vi "DiJian_1.vi"(8 "error in":errorcluster, 10 "地检1相位":i32, 11 "VISA资源名称":refnum<visa-resource-name>) -> (0 "错误输出":errorcluster, 2 "地检1相位输出":i32, 3 "VISA资源名称输出":refnum<visa-resource-name>)   [LabVIEW 2012]
uses:
  <vilib>/GPower/VIRegister/Library/Convert/ToDBL.vi
  <vilib>/GPower/VIRegister/Library/Convert/ToU16.vi
  <vilib>/GPower/VIRegister/Library/SubVIs/FindRegisterData.vi
  <vilib>/GPower/VIRegister/Library/SubVIs/ReadSub.vi
  <vilib>/GPower/VIRegister/Library/QManager/GetRegisterData.vi
  <vilib>/GPower/Error/Library/SetError.vi
  <vilib>/GPower/Error/Library/FilterCodes.vi
  <vilib>/GPower/Error/Library/Filter/FilterMulti.vi
  <vilib>/GPower/VIRegister/Library/QManager/QManagerAction.vi
  <vilib>/GPower/Error/Library/ErrorType.vi
  <vilib>/GPower/Error/Library/SplitAppended.vi
  <vilib>/GPower/Error/Library/SubVIs/ExplanationToError.vi
  <vilib>/GPower/VIRegister/Library/QManager/GetQName.vi
  <vilib>/GPower/VIRegister/Library/QManager/StartQManager.vi
  <vilib>/Utility/error.llb/Trim Whitespace.vi
  <vilib>/dlg_ctls.llb/Space Constant.vi
  <vilib>/Utility/error.llb/Error Code Database.vi
  <vilib>/GPower/Error/Library/SubVIs/SetStatus.vi
  <vilib>/GPower/Error/Library/AppendErrors.vi
  <vilib>/GPower/Error/Library/Append/AppendSingle.vi
  com/TONGXUN/write32.vi
  <vilib>/GPower/VIRegister/VIRegister.lvlib
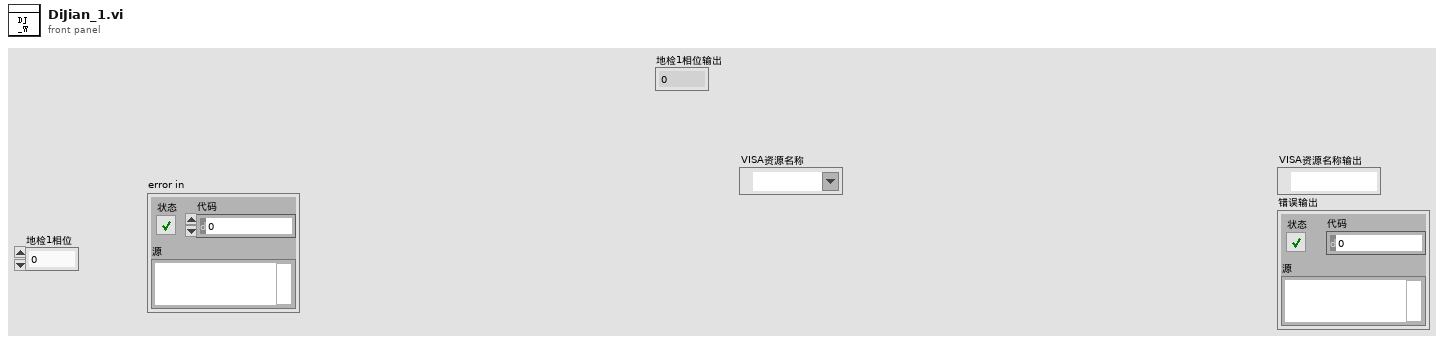
[diagram p1: front panel]
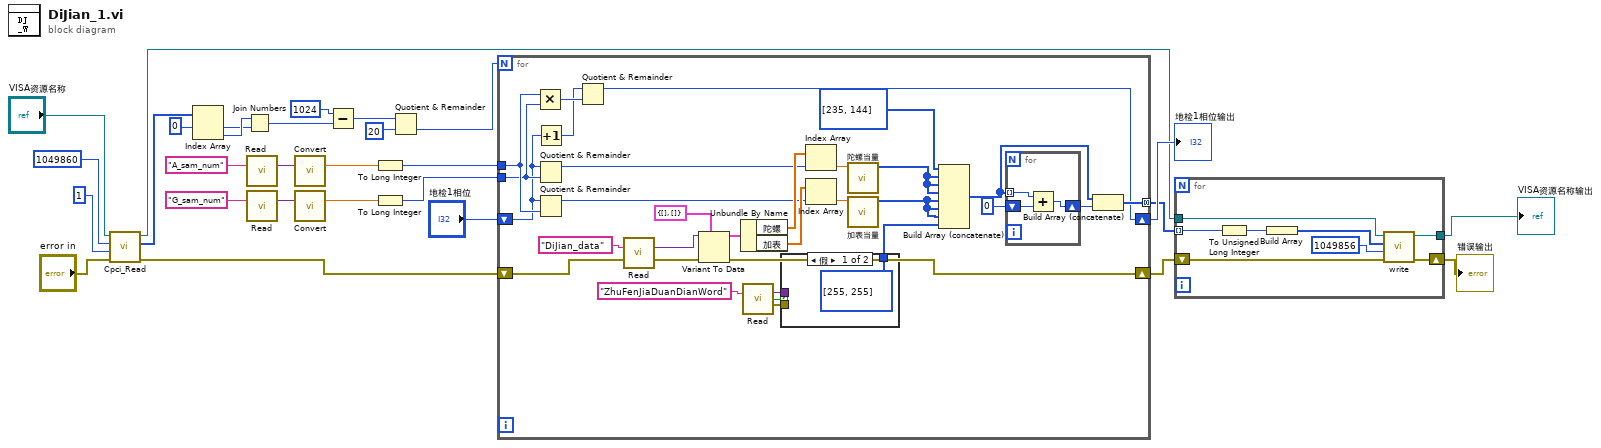
[diagram p0: block diagram]
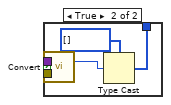
[diagram p2: hidden frame]
diagram:
  n1 = call "Cpci_Read.vi"("错误输入（无错误）"="error in", "u32_len"=1, "基地址"=u32 1049860, "VISA资源名称"="VISA资源名称") -> ("错误输出"=w1:errorcluster, "U8"=w9:u8[], "VISA资源名称输出"=w3:refnum<visa-resource-name>)  [unwired: 5 in]
  n2 = Index Array(array=w9, index #1=0 ("索引")) -> (element #1=w6:u8, element #2=w7:u8)  [unwired: 1 in]
  n3 = Join Numbers(hi=w7, lo=w6) -> ((hi.lo)=w12:u16)
  n4 = call <vilib>:"Read.vi"("Register name"="A_sam_num") -> ("Register value"=w22:variant)  [unwired: 11 in, 3 out]
  n5 = call <vilib>:"Read.vi"("Register name"="G_sam_num") -> ("Register value"=w19:variant)  [unwired: 11 in, 3 out]
  n6 = call-poly <vilib>:"Convert.vi"("Register value in"=w22) -> ("Register value out"=w23:dbl)  [unwired: 13 in, 1 out]
  n7 = call-poly <vilib>:"Convert.vi"("Register value in"=w19) -> ("Register value out"=w18:dbl)  [unwired: 13 in, 1 out]
  n8 = Subtract(x=u16 1024, y=w12) -> (x-y=w14:u16)
  n9 = To Long Integer(number=w23) -> (32bit integer=w20:i32)
  n10 = To Long Integer(number=w18) -> (32bit integer=w16:i32)
  n11 = Quotient & Remainder(x=w14, y=u16 20) -> (floor(x/y)=w5:u16)  [unwired: 1 out]
  n12 = for {
    N: w5 -> [_]
    tunnel: [w51] -> w4 mode=concatenating
    shift-right: [w50] -> w2
    shift-left: w1 -> [w49]
    shift-right: [w39] -> w24
    shift-left: "地检1相位" -> [w37]
    tunnel: w20 -> [w42]
    tunnel: w16 -> [w41]
    n13 = Multiply(x=w42, y=w41) -> (x*y=w40:i32)
    n14 = Increment(x=w37) -> (x+1=w38:i32)
    n15 = Quotient & Remainder(x=w37, y=w41) -> (x-y*floor(x/y)=w44:i32)  [unwired: 1 out]
    n16 = Quotient & Remainder(x=w37, y=w42) -> (x-y*floor(x/y)=w43:i32)  [unwired: 1 out]
    n17 = Quotient & Remainder(x=w38, y=w40) -> (x-y*floor(x/y)=w39:i32)  [unwired: 1 out]
    n18 = call <vilib>:"Read.vi"("Register name"="DiJian_data", "Error in"=w49) -> ("Register value"=w57:variant, "Error out"=w53:errorcluster)  [unwired: 10 in, 2 out]
    n19 = Variant To Data(error in=w53, type=cluster{"陀螺":dbl[], "加表":dbl[]} {"陀螺"=[], "加表"=[]} ("输入簇"), Variant=w57) -> (data=w58:cluster{"陀螺":dbl[], "加表":dbl[]}, error out=w50:errorcluster)
    n20 = Unbundle By Name(w58) -> ("陀螺"=w59:dbl[], "加表"=w60:dbl[])
    n21 = call <vilib>:"Read.vi"("Register name"="ZhuFenJiaDuanDianWord") -> ("Register value"=w34:variant, "Register value read?"=w32:bool, "Error out"=w35:errorcluster)  [unwired: 11 in, 1 out]
    n22 = case shown="假" w32 {
      tunnel: w35 -> [_ w66]
      tunnel: w34 -> [_ w65]
      tunnel: [u8[] [255, 255] ("反转的数组") w63] -> w33
      frame False {
      }
      frame True {
        n23 = call-poly <vilib>:"Convert.vi"("Register value in"=w65, "Error in"=w66) -> ("Register value out"=w64:u16)  [unwired: 12 in, 1 out]
        n24 = Type Cast(type=u8[] [] ("反转的数组"), x=w64) -> (*(type *) &x=w63:u8[])
      }
    }
    n25 = Index Array(array=w59, index=w44) -> (element=w47:dbl)
    n26 = Index Array(array=w60, index=w43) -> (element=w46:dbl)
    n27 = call "陀螺当量.vi"("x"=w47) -> ("子数组"=w31:u8[])  [unwired: 10 in]
    n28 = call "加表当量.vi"("x"=w46) -> ("子数组"=w30:u8[])  [unwired: 10 in]
    n29 = Build Array (concatenate)(u8[] [235, 144] ("数组"), w31, w31, w31, w30, w30, w30, w33) -> (w45:u8[])
    n30 = for {
      tunnel: w45 -> [w69] mode=indexing
      shift-right: [w67] -> w54
      shift-left: u8 0 ("y") -> [w68]
      n31 = Add(x=w69, y=w68) -> (x+y=w67:u8)
    }
    n32 = Build Array (concatenate)(w45, w54) -> (w51:u8[])
  }
  "地检1相位输出" <- w24
  n33 = for {
    tunnel: w4 -> [w77] mode=indexing
    tunnel: w3 -> [w76]
    tunnel: [w75] -> w28
    shift-right: [w73] -> w26
    shift-left: w2 -> [w74]
    n34 = To Unsigned Long Integer(number=w77) -> (unsigned 32bit integer=w70:u32)
    n35 = Build Array(w70) -> (w71:u32[])
    n36 = call-poly "write.vi"("error out"=w74, "起始地址"=u32 1049856, "U32"=w71, "VISA资源名称输入"=w76) -> ("error out 2"=w73:errorcluster, "VISA资源名称输出"=w75:refnum<visa-resource-name>)  [unwired: 6 in]
  }
  "VISA资源名称输出" <- w28
  "错误输出" <- w26
